vi "ZDataVIS_Index_Wavenames.vi"(11 "wave names":string[](array[string])) -> (3 "Index, Wavenames":string[][](table)=[["0", "'time.SA03008L.20190612.000014'\n"], ["1", "'temp.SA03008L.20190612.000014'\n"], ["2", "'B.SA03008L.20190612.000014'\n"], ["3", "'Brate.SA03008L.20190612.000014'\n"], ["4", "'Lockin1.SA03008L.20190612.000014'\n"], ["5", "'Lockin2.SA03008L.20190612.000014'\n"], ["6", "'Lockin3.SA03008L.20190612.000014'\n"], ["7", "'Lockin4.SA03008L.20190612.000014'\n"], ["8", "'Lockin5.SA03008L.20190612.000014'\n"], ["9", "'Lockin6.SA03008L.20190612.000014'\n"], ["10", "'AO1.SA03008L.20190612.000014'\n"], ["11", "'AO2.SA03008L.20190612.000014'\n"], ["12", "'AO3.SA03008L.20190612.000014'\n"], ["13", "'AO4.SA03008L.20190612.000014'\n"], ["14", "'AO5.SA03008L.20190612.000014'\n"], ["15", "'AO6.SA03008L.20190612.000014'\n"], ["16", "'AO7.SA03008L.20190612.000014'\n"], ["17", "'AO8.SA03008L.20190612.000014'\n"], ["", ""]])   [LabVIEW 2016]
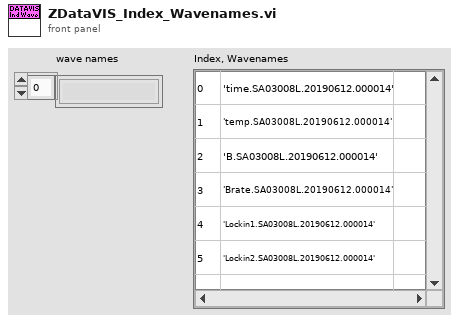
[diagram p1: front panel]
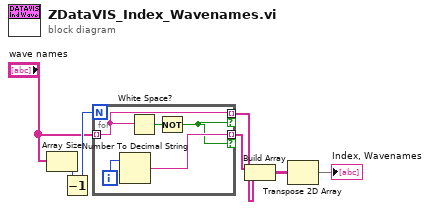
[diagram p0: block diagram]
diagram:
  n1 = Array Size(array="wave names") -> (size(s)=w5:i32)
  n2 = Decrement(x=w5) -> (x-1=w4:i32)
  n3 = for {
    N: w4 -> [_]
    tunnel: [w11] -> w7 mode=indexing if=w8
    tunnel: "wave names" -> [w9] mode=indexing
    tunnel: [w9] -> w1 mode=indexing if=w8
    i -> [w12]
    n4 = Number To Decimal String(number=w12) -> (decimal integer string=w11:string)  [unwired: 1 in]
    n5 = White Space?(1:w9) -> (0:w10:bool)
    n6 = Not(x=w10) -> (.not. x?=w8:bool)
  }
  n7 = Build Array(w7, w1) -> (w3:string[][])
  n8 = Transpose 2D Array(2D array=w3) -> (transposed array=→"Index, Wavenames":string[][])
